vi "ExpandTableIfNeeded.vi"(8 "error in":errorcluster, 9 "Table Size":cluster{"Row":i32, "Column":i32}, 10 "Table in":refnum<k24>) -> (0 "error out":errorcluster, 2 "Table out":refnum<k24>)   [LabVIEW 2009, in "ooCalc.lvclass"]
uses:
  ooCalc/ooCalc.lvclass
  C:/Projets/LAVAG/OpenOfficeRGT/AODL/DLLs/AODL.dll
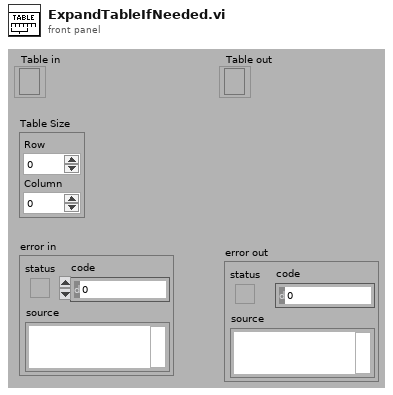
[diagram p1: front panel]
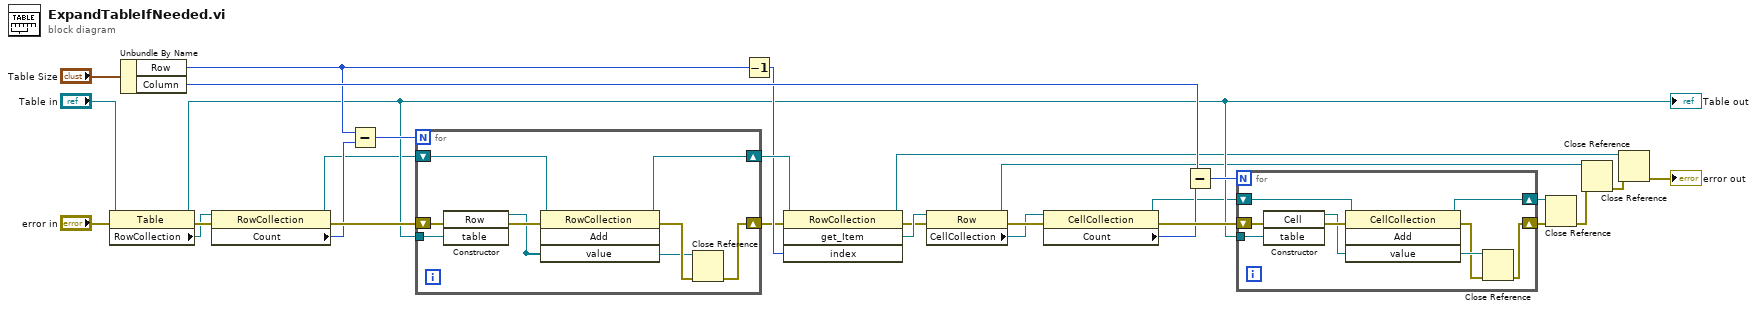
[diagram p0: block diagram]
diagram:
  n1 = property on="Property Node" class="Table"(reference="Table in", error in="error in") -> (reference out=w12:refnum<k24>, error out=w17:errorcluster, "RowCollection"=w14:refnum<k24>)
  "Table out" <- w12
  n2 = Unbundle By Name("Table Size") -> ("Row"=w20:i32, "Column"=w28:i32)
  n3 = property on="Property Node" class="RowCollection"(reference=w14, error in=w17) -> (reference out=w11:refnum<k24>, error out=w18:errorcluster, "Count"=w15:i32)
  n4 = Subtract(x=w20, y=w15) -> (x-y=w16:i32)
  n5 = for {
    N: w16 -> [_]
    shift-right: [w34] -> w27
    shift-left: w11 -> [w35]
    tunnel: w12 -> [w38]
    shift-right: [w32] -> w19
    shift-left: w18 -> [w37]
    n6 = constructor class="Row"(error in=w37, "table"=w38) -> (reference out=w31:refnum<k24>, error out=w36:errorcluster)  [unwired: 2 in, 2 out]
    n7 = invoke class="RowCollection" method="Add"(reference=w35, error in=w36, "value"=w31) -> (reference out=w34:refnum<k24>, error out=w33:errorcluster)  [unwired: 1 in, 2 out]
    n8 = Close Reference(reference=w31, error in (no error)=w33) -> (error out=w32:errorcluster)
  }
  n9 = Decrement(x=w20) -> (x-1=w21:i32)
  n10 = invoke class="RowCollection" method="get_Item"(reference=w27, error in=w19, "index"=w21) -> (reference out=w9:refnum<k24>, error out=w10:errorcluster, "get_Item"=w23:refnum<k24>)  [unwired: 1 in, 1 out]
  n11 = property on="Property Node" class="Row"(reference=w23, error in=w10) -> (reference out=w1:refnum<k24>, error out=w22:errorcluster, "CellCollection"=w8:refnum<k24>)
  n12 = property on="Property Node" class="CellCollection"(reference=w8, error in=w22) -> (reference out=w4:refnum<k24>, error out=w29:errorcluster, "Count"=w24:i32)
  n13 = Subtract(x=w28, y=w24) -> (x-y=w25:i32)
  n14 = for {
    N: w25 -> [_]
    shift-right: [w42] -> w7
    shift-left: w4 -> [w43]
    tunnel: w12 -> [w46]
    shift-right: [w39] -> w6
    shift-left: w29 -> [w45]
    n15 = constructor class="Cell"(error in=w45, "table"=w46) -> (reference out=w41:refnum<k24>, error out=w44:errorcluster)  [unwired: 2 in, 2 out]
    n16 = invoke class="CellCollection" method="Add"(reference=w43, error in=w44, "value"=w41) -> (reference out=w42:refnum<k24>, error out=w40:errorcluster)  [unwired: 1 in, 2 out]
    n17 = Close Reference(reference=w41, error in (no error)=w40) -> (error out=w39:errorcluster)
  }
  n18 = Close Reference(reference=w7, error in (no error)=w6) -> (error out=w3:errorcluster)
  n19 = Close Reference(reference=w1, error in (no error)=w3) -> (error out=w2:errorcluster)
  n20 = Close Reference(reference=w9, error in (no error)=w2) -> (error out=→"error out":errorcluster)
